vi "Compass_6532_Reading.vi"(2 "SRV In":string) -> (1 "Heading":dbl, 4 "SRV Out":string="169.254.0.10")   [LabVIEW 2009]
panel:
  out "Reply":string
  # "This LabVIEW item is deprecated.\n\nIt is believed to be unused and will be removed in a future version of SRV."
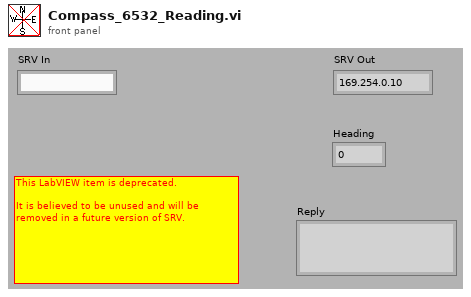
[diagram p1: front panel]
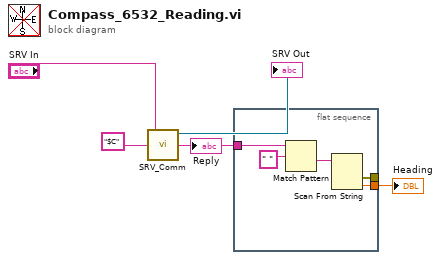
[diagram p0: block diagram]
diagram:
  n1 = call "SRV_Comm.vi"("Command Sent"="$C", "SRV In"="SRV In") -> ("Reply"=w5:string, "SRV Out"=→"SRV Out":refnum<k5>)  [unwired: 1 in, 1 out]
  "Reply" <- w5
  n2 = flat-sequence {
    tunnel: w5 -> [w10]
    tunnel: [w7] -> _
    tunnel: [w6] -> w1
    frame #0 {
      n3 = Match Pattern(string=w10, regular expression=" " ("Command Sent")) -> (after substring=w9:string)  [unwired: 1 in, 3 out]
      n4 = Scan From String(input string=w9) -> (error out=w7:errorcluster, output 1=w6:dbl)  [unwired: 4 in, 2 out]
    }
  }
  "Heading" <- w1
